vi "Do.vi"(8 "error in (no error)":errorcluster, 10 "Actor in":refnum<class "Actor.lvclass">, 11 "New Test Window Launched Msg":refnum<class "New Test Window Launched Msg.lvclass">) -> (0 "error out":errorcluster, 2 "Actor out":refnum<class "Actor.lvclass">)   [LabVIEW 2017, in "Test Application Controller.lvlib" / "New Test Window Launched Msg.lvclass"]
doc: "This VI delivers the message to the actor by calling the appropriate method(s) on the actor."
uses:
  New Test Window Launched Msg.lvclass
  D:/Career/Tesla/LabVIEW_Interview_Problem/Tesla Test Application/Test/Test Messages/Test Window Launched Msg/Test Window Launched Msg.lvclass
  <vilib>/ActorFramework/Actor/Actor.lvclass
  Test Application Controller/Test Application Controller.lvclass
  C:/Program Files (x86)/National Instruments/LabVIEW 2017/vi.lib/ActorFramework/Actor/Actor.lvclass
  Test/Test Messages/Test Window Launched Msg/Test Window Launched Msg.lvclass/Test Window Launched Msg.ctl
  Test/Test Messages/Test Window Launched Msg/Test Window Launched Msg.lvclass
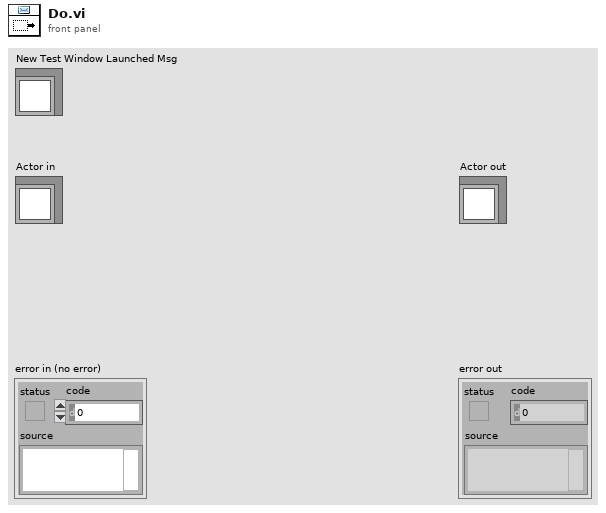
[diagram p1: front panel]
types:
  T1 = cluster{"Window Name":string, "VI Refnum":refnum<vi>}
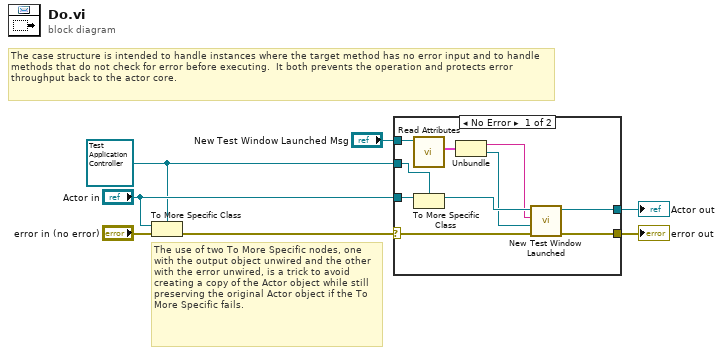
[diagram p0: block diagram]
diagram:
  w2 = refnum<class "Test Application Controller.lvclass"> refnum ("Actor in")
  # "The use of two To More Specific nodes, one with the output object unwired and the other with the error unwired, is a trick to avoid creating a copy of the Actor object while still preserving the original Actor object if the To More Specific fails."
  # "The case structure is intended to handle instances where the target method has no error input and to handle methods that do not check for error before executing.  It both prevents the operation and protects error throughput back to the actor core."
  n1 = To More Specific Class(target class=w2, reference="Actor in", error in="error in (no error)") -> (error out=w6:errorcluster)  [unwired: 1 out]
  n2 = case shown="No Error" w6 {
    selector: w6 -> [w15 w19]
    tunnel: [w17 w19] -> w5
    tunnel: [w16 w18] -> w4
    tunnel: "Actor in" -> [w14 w18]
    tunnel: w2 -> [w13 _]
    tunnel: "New Test Window Launched Msg" -> [w10 _]
    frame No Error {
      n3 = call "Read Attributes.vi"("Test Window Launched Msg"=w10) -> ("Payload"=w11:T1)  [unwired: 10 in]
      n4 = To More Specific Class(target class=w13, reference=w14) -> (specific class reference=w12:refnum<class "Test Application Controller.lvclass">)  [unwired: 1 in, 1 out]
      n5 = Unbundle(w11) -> ("Window Name"=w9:string, "VI Refnum"=w8:refnum<vi>)
      n6 = call "New Test Window Launched.vi"("error in (no error)"=w15, "VI Refnum"=w8, "Window Name"=w9, "Test Application Controller in"=w12) -> ("error out"=w17:errorcluster, "Test Application Controller out"=w16:refnum<class "Test Application Controller.lvclass">)  [unwired: 6 in]
    }
    frame Error {
      # "If type check fails, pass the original object out again."
    }
  }
  "error out" <- w5
  "Actor out" <- w4
